vi "stream_name_constant.vi"() -> (3 "log_stream_name":string="system.logger-log_stream")   [LabVIEW 2021, in "system.logging.lvclass"]
uses:
  system.logging.lvclass
  system.logging.lvclass/system.logging.ctl
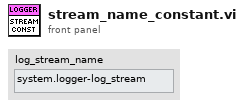
[diagram p1: front panel]
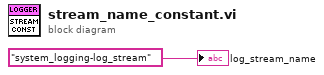
[diagram p0: block diagram]
diagram:
  "log_stream_name" <- "system_logging-log_stream"
